vi "AIClear.vi"(4 "error in (no error)":errorcluster, 7 "Params in":T1={"Manual Control"={"Rotation Control"={"Phase"=0.0, "A amp (0-120)"=75.0, "B amp (0-120)"=53.3, "mean freq  [MHz]\ndefault 39.99"=40.0, "freq difference [Hz]"=2.0, "Enable A"=TRUE, "Enable B"=TRUE}, "X piezo\n [nm]"=0.0, "Y peizo\n [nm]"=0.0, "-Z piezo\n [nm]"=5.012658227848101, "AOM0 \nPower"=0.2}, "Piezo Calibr"={"Px2Vx(AO)"=nan, "Py2Vy(AO)"=nan, "Pz2Vz(AO)"=nan, "Min Px"=nan, "Min Py"=nan, "Min Pz"=nan, "Max Px"=nan, "Max Py"=nan, "Max Pz"=nan}, "Instrument Calibr"={"TQGT"=[], "TetherCenter"={"TrapX_AO 0 [nm]"=nan, "TrapY_AO 0 [nm]"=nan, "TrapZ_AO 0 [nm]"=nan}, "XYZsignal baseline"={"Xsignal0"=0.0, "Ysignal0"=0.0, "Zsignal0"=0.0, "Zsig slope"=0.0, "Z bead0"=nan}, "S and P to Vs0"={"Vs0/P"=0.0, "Vs0/S"=0.0}, "Psi"=0.0, "ePS:eRL drift correlation"={"Interc P"=nan, "Slope P"=nan, "Interc S"=nan, "Slope S"=nan}, "Current piezo volt AO"={"Vpx_AO [V]"=nan, "Vpy_AO [V]"=nan, "Vpz_AO [V]"=nan}}, "Cylinder Calibr"={"ZStiff"=nan, "Zsens"=nan, "AngStiff"=nan, "XStiff"=nan, "Xsens"=nan, "MaxEllip"=nan, "YStiff"=nan, "Ysens"=nan, "FocalShift"=nan, "Sfz"=0.0, "1/Sz"=0.0, "Stau"=0.0, "Sfx"=0.0, "1/Sx"=0.0, "1/Sang"=0.0, "Sfy"=0.0, "1/Sy"=0.0, "1/focal"=0.0}, "DAQParams"={"Buffer size"=nan, "Scanning rate"=nan, "Average"=nan, "Sampling rate"=nan, "set dt"=nan}, "DAQ channel offsets"={"A0 [V]"=0.0, "D0 [V]"=0.0, "P0  [V]"=0.0, "S0 [V]"=0.0, "L0 [V]"=0.0, "R0 [V]"=0.0, "Vpx0 [V]"=0.0, "Vpy0 [V]"=0.0, "Vpz0 [V]"=0.0, "Vsum0 [V]"=0.0, "Vpx_AO0 [V]"=0.0, "Vpy_AO0 [V]"=0.0, "Vpz_AO0 [V]"=0.0}, "Z bead polynomial coeffs"=[nan, nan, nan, nan], "Skip button ref"=refnum, "z bead lookup table"={"z signal"=[], "z bead"=[]}, "SP->power Matrix"=[], "Ms2p"=[], "Mp2s"=[], "task in"="Oscilloscope2"} {"Instrument Calibr"."Psi" format="%#_2f"; "Manual Control"."Y peizo\n [nm]" scale=0.0..7000.0; "Manual Control"."AOM0 \nPower" scale=0.0..1.0; "Manual Control"."X piezo\n [nm]" scale=0.0..7000.0; "Manual Control"."Rotation Control"."freq difference [Hz]" step=0.5; "Manual Control"."Rotation Control"."mean freq  [MHz]\ndefault 39.99" min=0.0 step=0.01; "Manual Control"."Rotation Control"."B amp (0-120)" min=0.0 max=120.0 step=0.1; "Manual Control"."Rotation Control"."A amp (0-120)" min=0.0 max=120.0 step=0.1; "Manual Control"."Rotation Control"."Phase" scale=0.0..360.0; "Manual Control"."-Z piezo\n [nm]" scale=1000.0..7000.0}) -> (0 "error out":errorcluster, 3 "Params out":T1={"Manual Control"={"Rotation Control"={"Phase"=0.0, "A amp (0-120)"=75.0, "B amp (0-120)"=53.3, "mean freq  [MHz]\ndefault 39.99"=40.0, "freq difference [Hz]"=2.0, "Enable A"=TRUE, "Enable B"=TRUE}, "X piezo\n [nm]"=0.0, "Y peizo\n [nm]"=0.0, "-Z piezo\n [nm]"=5.012658227848101, "AOM0 \nPower"=0.2}, "Piezo Calibr"={"Px2Vx(AO)"=nan, "Py2Vy(AO)"=nan, "Pz2Vz(AO)"=nan, "Min Px"=nan, "Min Py"=nan, "Min Pz"=nan, "Max Px"=nan, "Max Py"=nan, "Max Pz"=nan}, "Instrument Calibr"={"TQGT"=[], "TetherCenter"={"TrapX_AO 0 [nm]"=nan, "TrapY_AO 0 [nm]"=nan, "TrapZ_AO 0 [nm]"=nan}, "XYZsignal baseline"={"Xsignal0"=0.0, "Ysignal0"=0.0, "Zsignal0"=0.0, "Zsig slope"=0.0, "Z bead0"=nan}, "S and P to Vs0"={"Vs0/P"=0.0, "Vs0/S"=0.0}, "Psi"=0.0, "ePS:eRL drift correlation"={"Interc P"=nan, "Slope P"=nan, "Interc S"=nan, "Slope S"=nan}, "Current piezo volt AO"={"Vpx_AO [V]"=nan, "Vpy_AO [V]"=nan, "Vpz_AO [V]"=nan}}, "Cylinder Calibr"={"ZStiff"=nan, "Zsens"=nan, "AngStiff"=nan, "XStiff"=nan, "Xsens"=nan, "MaxEllip"=nan, "YStiff"=nan, "Ysens"=nan, "FocalShift"=nan, "Sfz"=0.0, "1/Sz"=0.0, "Stau"=0.0, "Sfx"=0.0, "1/Sx"=0.0, "1/Sang"=0.0, "Sfy"=0.0, "1/Sy"=0.0, "1/focal"=0.0}, "DAQParams"={"Buffer size"=nan, "Scanning rate"=nan, "Average"=nan, "Sampling rate"=nan, "set dt"=nan}, "DAQ channel offsets"={"A0 [V]"=0.0, "D0 [V]"=0.0, "P0  [V]"=0.0, "S0 [V]"=0.0, "L0 [V]"=0.0, "R0 [V]"=0.0, "Vpx0 [V]"=0.0, "Vpy0 [V]"=0.0, "Vpz0 [V]"=0.0, "Vsum0 [V]"=0.0, "Vpx_AO0 [V]"=0.0, "Vpy_AO0 [V]"=0.0, "Vpz_AO0 [V]"=0.0}, "Z bead polynomial coeffs"=[nan, nan, nan, nan], "Skip button ref"=refnum, "z bead lookup table"={"z signal"=[], "z bead"=[]}, "SP->power Matrix"=[], "Ms2p"=[], "Mp2s"=[], "task in"="Oscilloscope2"} {"Instrument Calibr"."Psi" format="%#_2f"; "Manual Control"."Y peizo\n [nm]" scale=0.0..7000.0; "Manual Control"."AOM0 \nPower" scale=0.0..1.0; "Manual Control"."X piezo\n [nm]" scale=0.0..7000.0; "Manual Control"."Rotation Control"."freq difference [Hz]" step=0.5; "Manual Control"."Rotation Control"."mean freq  [MHz]\ndefault 39.99" min=0.0 step=0.01; "Manual Control"."Rotation Control"."B amp (0-120)" min=0.0 max=120.0 step=0.1; "Manual Control"."Rotation Control"."A amp (0-120)" min=0.0 max=120.0 step=0.1; "Manual Control"."Rotation Control"."Phase" scale=0.0..360.0; "Manual Control"."-Z piezo\n [nm]" scale=1000.0..7000.0})   [LabVIEW 2017, in "Data aquisition.lvlib"]
uses:
  Data aquisition.lvlib
  Initialization/Param.ctl
  Initialization/ManualCtrl.ctl
  Initialization/Initialization.lvlib
  Initialization/CylinderCalibrNew.ctl
  <vilib>/Analysis/Matrix/Datatypes/RealMatrix.ctl
  <vilib>/Analysis/Matrix/NI_Matrix.lvlib
  SignalConversion/DAQChannelOffsets.ctl
  SignalConversion/SignalConverson.lvlib
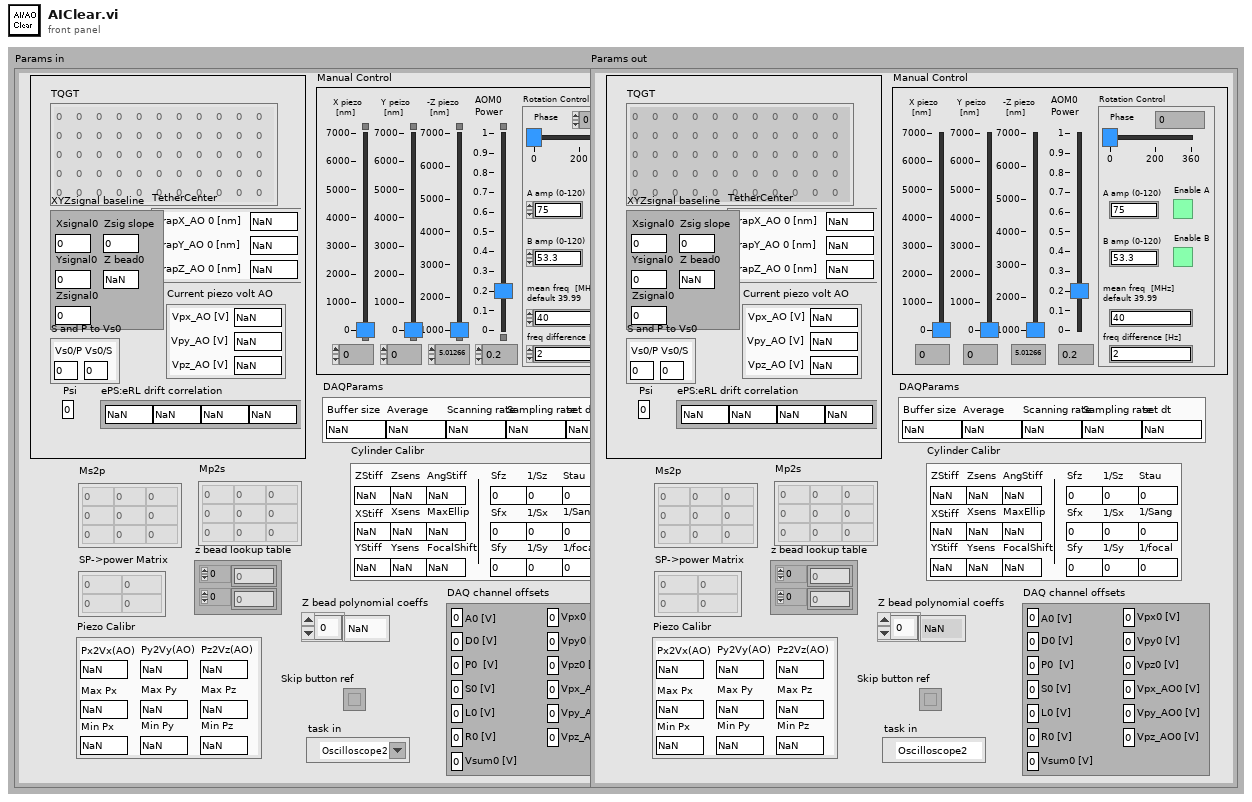
[diagram p1: front panel]
types:
  T1 = typedef "Param.ctl" = cluster{"Manual Control":T2, "Piezo Calibr":cluster{"Px2Vx(AO)":dbl, "Py2Vy(AO)":dbl, "Pz2Vz(AO)":dbl, "Min Px":dbl, "Min Py":dbl, "Min Pz":dbl, "Max Px":dbl, "Max Py":dbl, "Max Pz":dbl}, "Instrument Calibr":cluster{"TQGT":dbl[][], "TetherCenter":cluster{"TrapX_AO 0 [nm]":dbl, "TrapY_AO 0 [nm]":dbl, "TrapZ_AO 0 [nm]":dbl}, "XYZsignal baseline":cluster{"Xsignal0":dbl, "Ysignal0":dbl, "Zsignal0":dbl, "Zsig slope":dbl, "Z bead0":dbl}, "S and P to Vs0":cluster{"Vs0/P":dbl, "Vs0/S":dbl}, "Psi":dbl, "ePS:eRL drift correlation":cluster{"Interc P":dbl, "Slope P":dbl, "Interc S":dbl, "Slope S":dbl}, "Current piezo volt AO":cluster{"Vpx_AO [V]":dbl, "Vpy_AO [V]":dbl, "Vpz_AO [V]":dbl}}, "Cylinder Calibr":T3, "DAQParams":cluster{"Buffer size":dbl, "Scanning rate":dbl, "Average":dbl, "Sampling rate":dbl, "set dt":dbl}, "DAQ channel offsets":T4, "Z bead polynomial coeffs":dbl[], "Skip button ref":refnum<vi>, "z bead lookup table":cluster{"z signal":dbl[], "z bead":dbl[]}, "SP->power Matrix":T5, "Ms2p":T5, "Mp2s":T5, "task in":refnum<k21>}
  T2 = typedef "Initialization.lvlib/ManualCtrl.ctl" = cluster{"Rotation Control":cluster{"Phase":dbl, "A amp (0-120)":dbl, "B amp (0-120)":dbl, "mean freq  [MHz]\ndefault 39.99":dbl, "freq difference [Hz]":dbl, "Enable A":bool, "Enable B":bool}, "X piezo\n [nm]":dbl, "Y peizo\n [nm]":dbl, "-Z piezo\n [nm]":dbl, "AOM0 \nPower":dbl}
  T3 = typedef "Initialization.lvlib/CylinderCalibrNew.ctl" = cluster{"ZStiff":dbl, "Zsens":dbl, "AngStiff":dbl, "XStiff":dbl, "Xsens":dbl, "MaxEllip":dbl, "YStiff":dbl, "Ysens":dbl, "FocalShift":dbl, "Sfz":dbl, "1/Sz":dbl, "Stau":dbl, "Sfx":dbl, "1/Sx":dbl, "1/Sang":dbl, "Sfy":dbl, "1/Sy":dbl, "1/focal":dbl}
  T4 = typedef "SignalConverson.lvlib/DAQChannelOffsets.ctl" = cluster{"A0 [V]":dbl, "D0 [V]":dbl, "P0  [V]":dbl, "S0 [V]":dbl, "L0 [V]":dbl, "R0 [V]":dbl, "Vpx0 [V]":dbl, "Vpy0 [V]":dbl, "Vpz0 [V]":dbl, "Vsum0 [V]":dbl, "Vpx_AO0 [V]":dbl, "Vpy_AO0 [V]":dbl, "Vpz_AO0 [V]":dbl}
  T5 = typedef "NI_Matrix.lvlib/RealMatrix.ctl" = dbl[][]
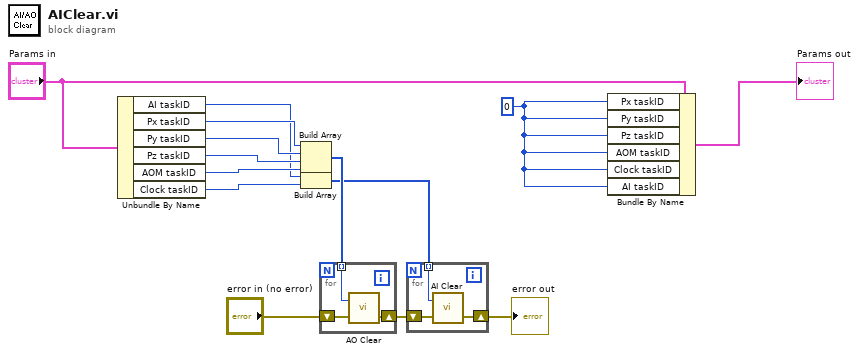
[diagram p0: block diagram]
diagram:
  w2 = u32 0 ("TaskIDs.DAQ tasks.Pu taskID")
  n1 = Unbundle By Name("Params in") -> ("AI taskID"=w8:u32, "Px taskID"=w14:u32, "Py taskID"=w13:u32, "Pz taskID"=w12:u32, "AOM taskID"=w11:u32, "Clock taskID"=w1:u32)
  n2 = Build Array(w14, w13, w12, w11) -> (w10:u32[])
  n3 = Build Array(w8, w1) -> (w7:u32[])
  n4 = for {
    tunnel: w10 -> [w17] mode=indexing
    shift-right: [w15] -> w6
    shift-left: "error in (no error)" -> [w16]
    n5 = call <vilib>:"AO Clear.vi"("error in (no error)"=w16, "taskID in"=w17) -> ("error out"=w15:errorcluster)  [unwired: 4 in, 1 out]
  }
  n6 = for {
    tunnel: w7 -> [w18] mode=indexing
    shift-right: [w19] -> w5
    shift-left: w6 -> [w20]
    n7 = call <vilib>:"AI Clear.vi"("error in (no error)"=w20, "taskID in"=w18) -> ("error out"=w19:errorcluster)  [unwired: 4 in, 1 out]
  }
  "error out" <- w5
  n8 = Bundle By Name(cluster="Params in", "Px taskID"=w2, "Py taskID"=w2, "Pz taskID"=w2, "AOM taskID"=w2, "Clock taskID"=w2, "AI taskID"=w2) -> (→"Params out":T1)
